vi "Close.vi"(8 "error in (no error)":errorcluster, 11 "Logger in":refnum<class "Logger.lvclass">) -> (0 "error out":errorcluster, 3 "Logger out":refnum<class "Logger.lvclass">)   [LabVIEW 2019, in "Logger.lvclass"]
uses:
  Logger.lvclass
  Logger.lvclass/Logger.ctl
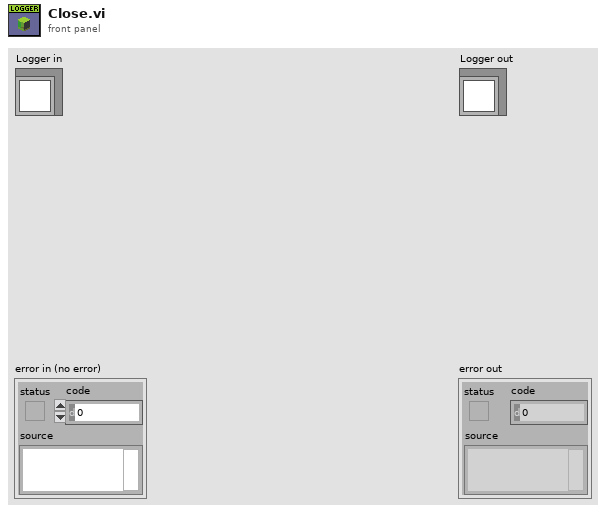
[diagram p1: front panel]
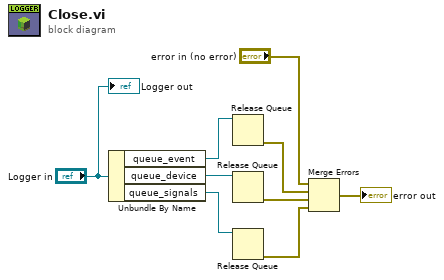
[diagram p0: block diagram]
diagram:
  n1 = Unbundle By Name("Logger in") -> ("queue_event"=w8:refnum<queue>, "queue_device"=w7:refnum<queue>, "queue_signals"=w6:refnum<queue>)
  n2 = Release Queue(queue=w8) -> (error out=w2:errorcluster)  [unwired: 2 in, 2 out]
  n3 = Release Queue(queue=w7) -> (error out=w3:errorcluster)  [unwired: 2 in, 2 out]
  n4 = Release Queue(queue=w6) -> (error out=w4:errorcluster)  [unwired: 2 in, 2 out]
  n5 = Merge Errors("error in (no error)", w2, w3, w4) -> (→"error out":errorcluster)
  "Logger out" <- "Logger in"
